vi "_AllThings.vi"   [LabVIEW 2024]
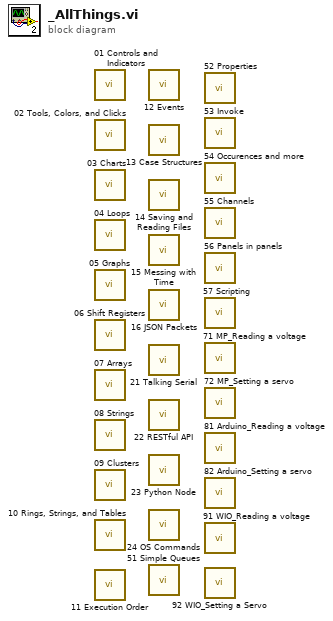
[diagram p0: block diagram]
diagram:
  n1 = call <userlib>:"01 Controls and Indicators.vi"() -> ()  [unwired: 12 in]
  n2 = call <userlib>:"02 Tools, Colors, and Clicks.vi"() -> ()  [unwired: 12 in]
  n3 = call <userlib>:"03 Charts.vi"() -> ()  [unwired: 12 in]
  n4 = call <userlib>:"04 Loops.vi"() -> ()  [unwired: 12 in]
  n5 = call <userlib>:"05 Graphs.vi"() -> ()  [unwired: 12 in]
  n6 = call <userlib>:"06 Shift Registers.vi"() -> ()  [unwired: 12 in]
  n7 = call <userlib>:"07 Arrays.vi"() -> ()  [unwired: 12 in]
  n8 = call <userlib>:"08 Strings.vi"() -> ()  [unwired: 12 in]
  n9 = call <userlib>:"09 Clusters.vi"() -> ()  [unwired: 12 in]
  n10 = call <userlib>:"10 Rings, Strings, and Tables.vi"() -> ()  [unwired: 12 in]
  n11 = call <userlib>:"11 Execution Order.vi"() -> ()  [unwired: 12 in]
  n12 = call <userlib>:"12 Events.vi"() -> ()  [unwired: 12 in]
  n13 = call <userlib>:"13 Case Structures.vi"() -> ()  [unwired: 12 in]
  n14 = call <userlib>:"14 Saving and Reading Files.vi"() -> ()  [unwired: 12 in]
  n15 = call <userlib>:"15 Messing with Time.vi"() -> ()  [unwired: 12 in]
  n16 = call <userlib>:"16 JSON Packets.vi"() -> ()  [unwired: 12 in]
  n17 = call <userlib>:"21 Talking Serial.vi"() -> ()  [unwired: 12 in]
  n18 = call <userlib>:"22 RESTful API.vi"() -> ()  [unwired: 12 in]
  n19 = call <userlib>:"23 Python Node.vi"() -> ()  [unwired: 12 in]
  n20 = call <userlib>:"24 OS Commands.vi"() -> ()  [unwired: 12 in]
  n21 = call <userlib>:"51 Simple Queues.vi"() -> ()  [unwired: 12 in]
  n22 = call <userlib>:"52 Properties.vi"() -> ()  [unwired: 12 in]
  n23 = call <userlib>:"53 Invoke.vi"() -> ()  [unwired: 12 in]
  n24 = call <userlib>:"54 Occurences and more.vi"() -> ()  [unwired: 12 in]
  n25 = call <userlib>:"55 Channels.vi"() -> ()  [unwired: 12 in]
  n26 = call <userlib>:"56 Panels in panels.vi"() -> ()  [unwired: 12 in]
  n27 = call <userlib>:"57 Scripting.vi"() -> ()  [unwired: 12 in]
  n28 = call <userlib>:"71 MP_Reading a voltage.vi"() -> ()  [unwired: 12 in]
  n29 = call <userlib>:"72 MP_Setting a servo.vi"() -> ()  [unwired: 12 in]
  n30 = call <userlib>:"81 Arduino_Reading a voltage.vi"() -> ()  [unwired: 12 in]
  n31 = call <userlib>:"82 Arduino_Setting a servo.vi"() -> ()  [unwired: 12 in]
  n32 = call <userlib>:"91 WIO_Reading a voltage.vi"() -> ()  [unwired: 12 in]
  n33 = call <userlib>:"92 WIO_Setting a Servo.vi"() -> ()  [unwired: 12 in]
